vi "random_access_subpattern.vi"(6 "ellipsoid parameter cluster":T1={"a"=0.0, "b"=0.125, "c"=0.5, "d"=0.015625, "e"=0.5, "k"=50, "width"=0.0} {"a" format="%.16g"; "b" format="%.16g"; "c" format="%.16g"; "d" format="%.16g"}, 8 "rotation cluster in":T2={"ellipsoid"={"counter"=0, "~x n"=0.999969482421875, "~y n"=0.0, "~z n"=5.0, "amp 0"=0.0}} {"ellipsoid"."amp 0" format="%.16g"; "ellipsoid"."~y n" format="%.16g"; "ellipsoid"."~x n" format="%.16g"}, 11 "scan points cluster in":T3) -> (0 "rotation cluster out":T2={"ellipsoid"={"counter"=0, "~x n"=0.999969482421875, "~y n"=0.0, "~z n"=5.0, "amp 0"=0.0}} {"ellipsoid"."amp 0" format="%.16g"; "ellipsoid"."~y n" format="%.16g"; "ellipsoid"."~x n" format="%.16g"}, 3 "scan points cluster out":T3)   [LabVIEW 2010]
uses:
  scan_points_cluster.ctl
  anti-photo-bleaching_rotation_cluster.ctl
  ellipsoid_parameters_cluster.ctl
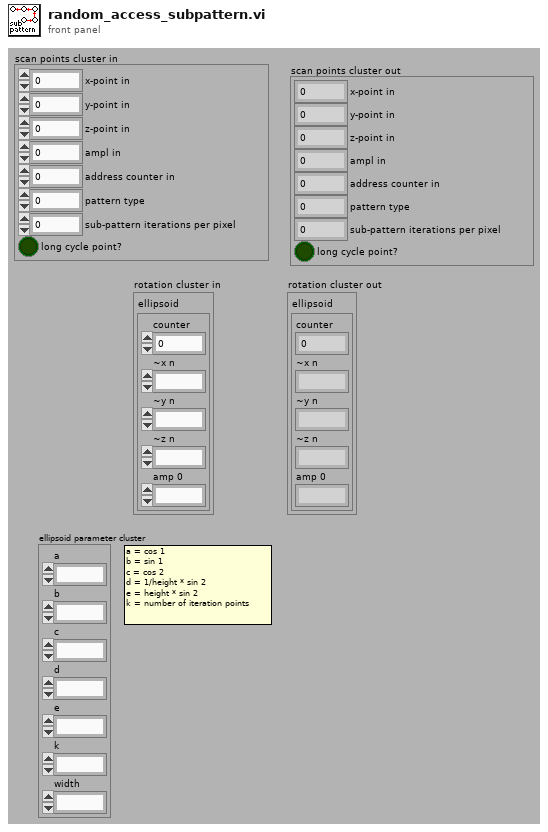
[diagram p1: front panel]
types:
  T1 = typedef "ellipsoid_parameters_cluster.ctl" = cluster{"a":fxp<+/-,16,1>, "b":fxp<+/-,16,1>, "c":fxp<+/-,16,1>, "d":fxp<+/-,16,1>, "e":fxp<+/-,24,16>, "k":u16, "width":fxp<+,16,16>}
  T2 = typedef "anti-photo-bleaching_rotation_cluster.ctl" = cluster{"ellipsoid":cluster{"counter":u16, "~x n":fxp<+/-,16,1>, "~y n":fxp<+/-,16,1>, "~z n":fxp<+/-,32,16>, "amp 0":fxp<+/-,16,1>}}
  T3 = typedef "scan_points_cluster.ctl" = cluster{"x-point in":i32, "y-point in":i32, "z-point in":i32, "ampl in":u16, "address counter in":i32, "pattern type":i8, "sub-pattern iterations per pixel":u16, "long cycle point?":bool}
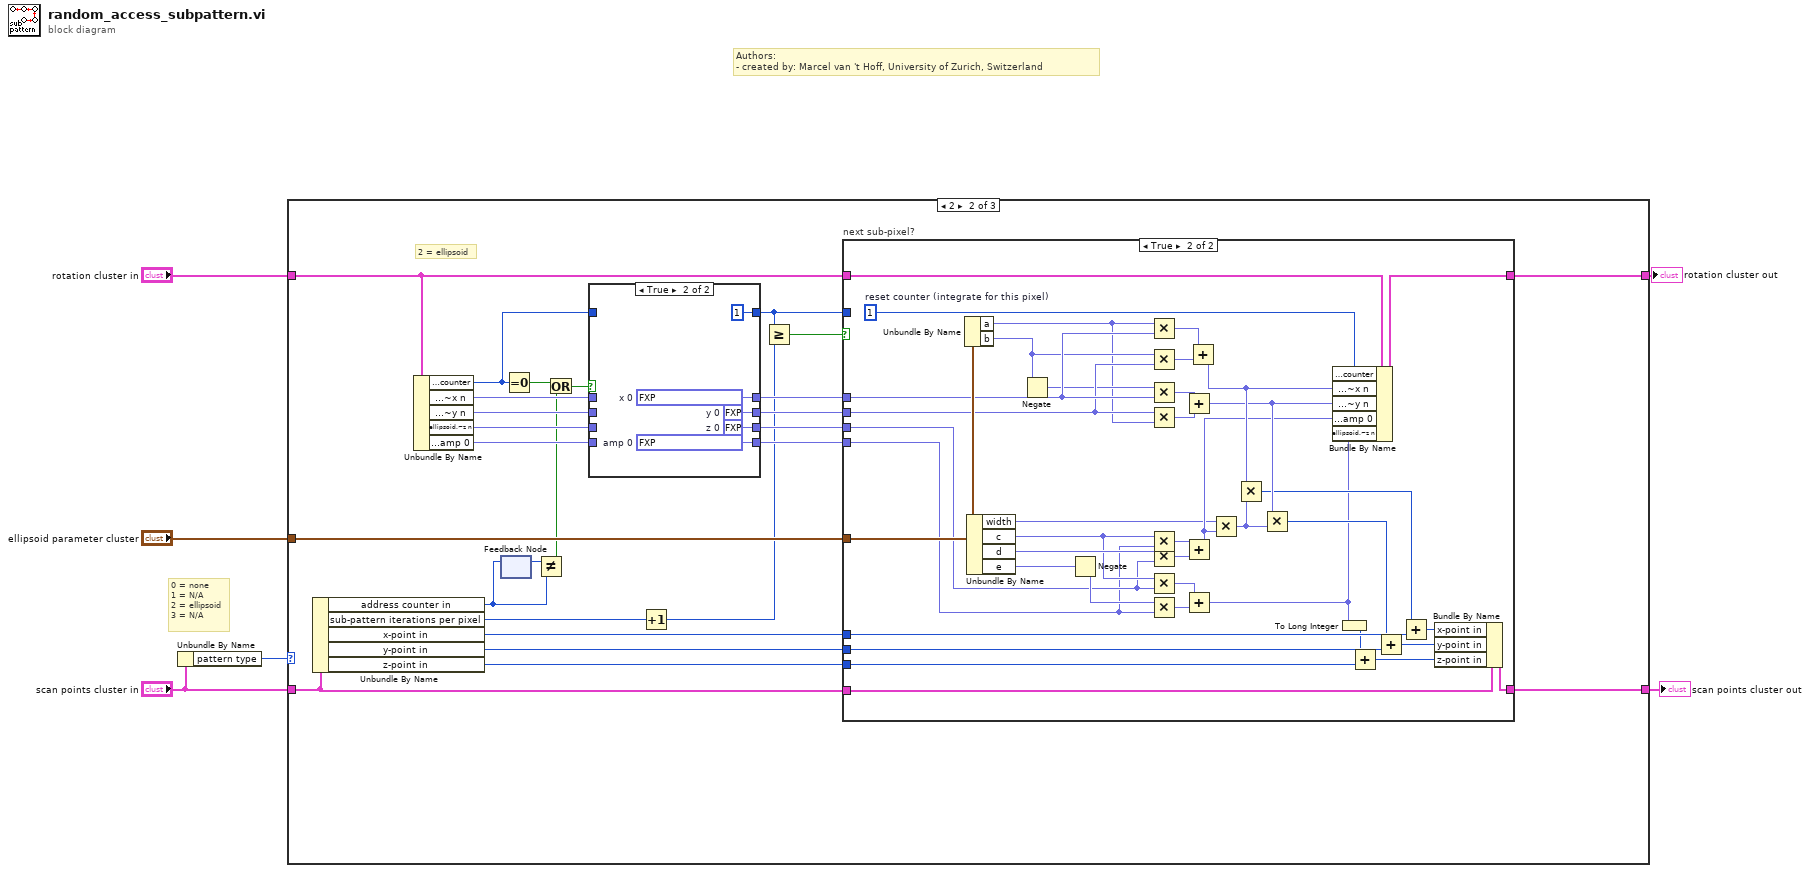
[diagram p0: block diagram]
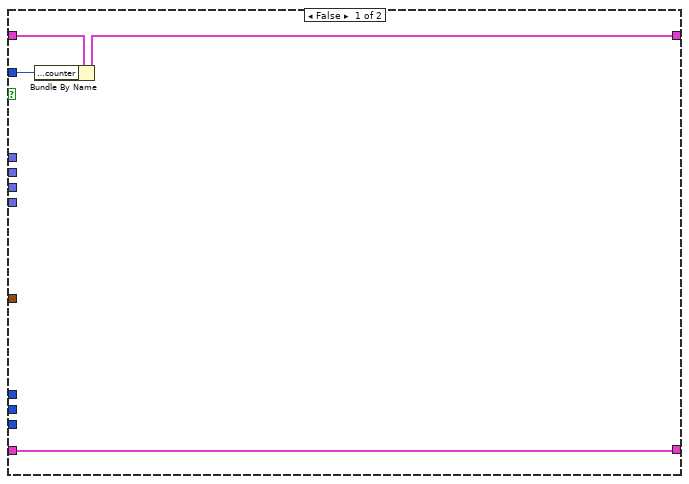
[diagram p3: hidden frame]
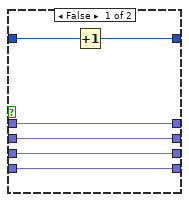
[diagram p4: hidden frame]
diagram:
  # "0 = none\n1 = N/A\n2 = ellipsoid\n3 = N/A"
  # "Authors: \n- created by: Marcel van 't Hoff, University of Zurich, Switzerland"
  n1 = Unbundle By Name("scan points cluster in") -> ("pattern type"=w1:i8)
  n2 = case shown="2" w1 {
    tunnel: "rotation cluster in" -> [w8 w27 w91]
    tunnel: [w8 w26 w91] -> w5
    tunnel: [w7 w22 w90] -> w4
    tunnel: "scan points cluster in" -> [w7 w23 w90]
    tunnel: "ellipsoid parameter cluster" -> [_ w34 _]
    frame 0, Default {
      # "0 = none"
    }
    frame 2 {
      # "2 = ellipsoid"
      n3 = Unbundle By Name(w23) -> ("address counter in"=w17:i32, "sub-pattern iterations per pixel"=w12:u16, "x-point in"=w21:i32, "y-point in"=w19:i32, "z-point in"=w20:i32)
      n4 = Unbundle By Name(w27) -> ("ellipsoid.counter"=w16:u16, "ellipsoid.~x n"=w33:fxp<+/-,16,1>, "ellipsoid.~y n"=w32:fxp<+/-,16,1>, "ellipsoid.~z n"=w31:fxp<+/-,32,16>, "ellipsoid.amp 0"=w30:fxp<+/-,16,1>)
      n5 = feedback-in #1(w17) -> ()
      n6 = feedback #1() -> (w18:i32)  [unwired: 1 in]
      n7 = Equal To 0?(x=w16) -> (x = 0?=w14:bool)
      n8 = Not Equal?(x=w18, y=w17) -> (x != y?=w15:bool)
      n9 = Or(x=w14, y=w15) -> (x .or. y?=w13:bool)
      n10 = case shown="True" w13 {
        tunnel: w33 -> [w84 _]
        tunnel: w32 -> [w83 _]
        tunnel: w31 -> [w82 _]
        tunnel: w30 -> [w81 _]
        tunnel: [w84 w89] -> w29
        tunnel: [w83 w88] -> w28
        tunnel: [w82 w86] -> w25
        tunnel: [w81 w87] -> w24
        tunnel: w16 -> [w80 _]
        tunnel: [w79 u16 1] -> w11
        frame False {
          n11 = Increment(x=w80) -> (x+1=w79:u16)
        }
        frame True {
          w86 = fxp<+/-,32,16> 0.0  # z 0
          w87 = fxp<+/-,16,1> 0.999969482421875  # amp 0
          w88 = fxp<+/-,16,1> 0.0  # y 0
          w89 = fxp<+/-,16,1> 0.999969482421875  # x 0
        }
      }
      n12 = Increment(x=w12) -> (x+1=w9:u16)
      n13 = Greater Or Equal?(x=w11, y=w9) -> (x >= y?=w10:bool)
      n14 = case "next sub-pixel?" shown="True" w10 {
        tunnel: w34 -> [_ w78]
        tunnel: w29 -> [_ w77]
        tunnel: w28 -> [_ w76]
        tunnel: w27 -> [w36 w72]
        tunnel: [w35 w71] -> w26
        tunnel: w25 -> [_ w53]
        tunnel: w24 -> [_ w52]
        tunnel: w23 -> [w38 w51]
        tunnel: [w38 w50] -> w22
        tunnel: w21 -> [_ w49]
        tunnel: w20 -> [_ w44]
        tunnel: w19 -> [_ w43]
        tunnel: w11 -> [w37 _]
        frame False {
          n15 = Bundle By Name(cluster=w36, "ellipsoid.counter"=w37) -> (w35:T2)
        }
        frame True {
          w40 = u16 1  # reset counter (integrate for this pixel)
          n16 = Unbundle By Name(w78) -> ("a"=w66:fxp<+/-,16,1>, "b"=w68:fxp<+/-,16,1>)
          n17 = Unbundle By Name(w78) -> ("width"=w54:fxp<+,16,16>, "c"=w58:fxp<+/-,16,1>, "d"=w62:fxp<+/-,16,1>, "e"=w60:fxp<+/-,24,16>)
          n18 = Negate(x=w68) -> (-x=w67:fxp<+/-,17,2>)
          n19 = Negate(x=w60) -> (-x=w59:fxp<+/-,25,17>)
          n20 = Multiply(x=w66, y=w77) -> (x*y=w70:fxp<+/-,32,2>)
          n21 = Multiply(x=w68, y=w76) -> (x*y=w69:fxp<+/-,32,2>)
          n22 = Multiply(x=w67, y=w77) -> (x*y=w64:fxp<+/-,31,1>)
          n23 = Multiply(x=w76, y=w66) -> (x*y=w65:fxp<+/-,32,2>)
          n24 = Multiply(x=w58, y=w52) -> (x*y=w63:fxp<+/-,32,2>)
          n25 = Multiply(x=w62, y=w53) -> (x*y=w61:fxp<+/-,48,17>)
          n26 = Multiply(x=w58, y=w53) -> (x*y=w56:fxp<+/-,48,17>)
          n27 = Multiply(x=w59, y=w52) -> (x*y=w57:fxp<+/-,39,16>)
          n28 = Add(x=w64, y=w65) -> (x+y=w74:fxp<+/-,16,1>)
          n29 = Add(x=w63, y=w61) -> (x+y=w73:fxp<+/-,16,1>)
          n30 = Add(x=w56, y=w57) -> (x+y=w45:fxp<+/-,32,16>)
          n31 = Add(x=w70, y=w69) -> (x+y=w75:fxp<+/-,16,1>)
          n32 = Multiply(x=w54, y=w73) -> (x*y=w55:fxp<+/-,32,17>)
          n33 = Multiply(x=w75, y=w55) -> (x*y=w46:i32)
          n34 = Multiply(x=w74, y=w55) -> (x*y=w47:i32)
          n35 = Bundle By Name(cluster=w72, "ellipsoid.counter"=w40, "ellipsoid.~x n"=w75, "ellipsoid.~y n"=w74, "ellipsoid.amp 0"=w73, "ellipsoid.~z n"=w45) -> (w71:T2)
          n36 = To Long Integer(number=w45) -> (32bit integer=w39:i32)
          n37 = Add(x=w39, y=w44) -> (x+y=w41:i32)
          n38 = Add(x=w47, y=w43) -> (x+y=w42:i32)
          n39 = Add(x=w46, y=w49) -> (x+y=w48:i32)
          n40 = Bundle By Name(cluster=w51, "x-point in"=w48, "y-point in"=w42, "z-point in"=w41) -> (w50:T3)
        }
      }
    }
    frame 3 {
      # "3 = N/A"
    }
  }
  "scan points cluster out" <- w4
  "rotation cluster out" <- w5
